vi "Scale Values.vi"(8 "error in (no error)":errorcluster, 10 "Values":dbl[](array[numeric]), 11 "VolatusScaling in":refnum<class "Scaling.lvclass">) -> (0 "error out":errorcluster, 2 "Scaled Values":dbl[](array[numeric]), 3 "VolatusScaling out":refnum<class "Scaling.lvclass">)   [LabVIEW 2020, in "VolatusData.lvlib" / "Scaling.lvclass"]
uses:
  Scaling.lvclass
  Scaling.lvclass/Scaling.ctl
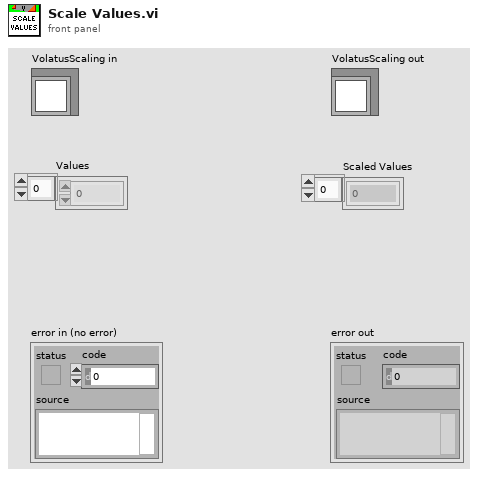
[diagram p1: front panel]
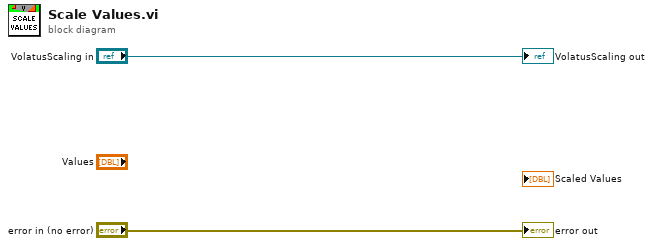
[diagram p0: block diagram]
diagram:
  "error out" <- "error in (no error)"
  "VolatusScaling out" <- "VolatusScaling in"
